vi "TKPS252XG Read Current-Voltage24.vi"(6 "error in (no error)":errorcluster, 8 "channel (ch1:0)":u16(ring) items=["channel 1", "channel 2", "channel 3"], 9 "VISA session":refnum<visa-resource-name>) -> (0 "error out":errorcluster, 1 "voltage limit":dbl format="%.4f", 2 "actual output voltage":dbl format="%.4f", 3 "dup VISA session":refnum<visa-resource-name>, 4 "current limit":dbl format="%.3f", 5 "actual output current":dbl format="%.4f", 7 "output":bool)   [LabVIEW 2024]
doc: "This vi queries the power supply for the current and voltage limits, the actual current and voltage being output, and the output state (on/off)."
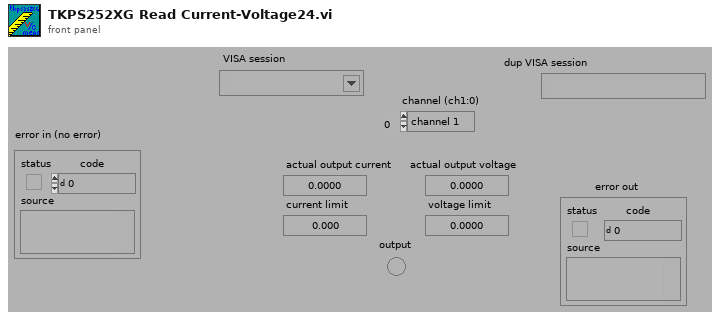
[diagram p1: front panel]
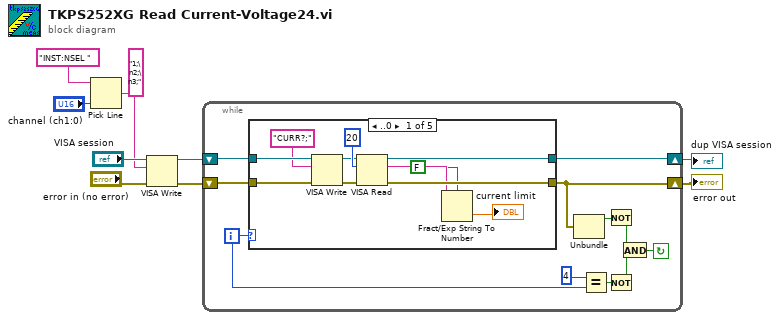
[diagram p0: block diagram]
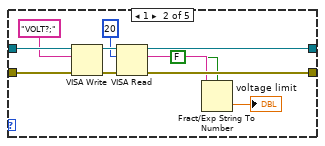
[diagram p2: hidden frame]
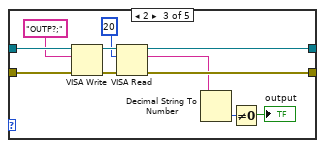
[diagram p3: hidden frame]
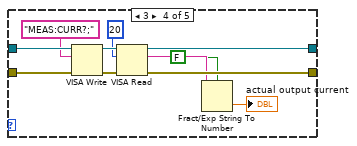
[diagram p4: hidden frame]
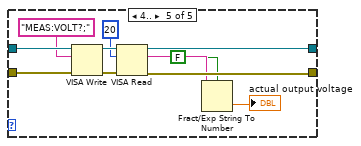
[diagram p5: hidden frame]
diagram:
  n1 = Pick Line(string ("")="INST:NSEL " ("VI name"), multi-line string="1;\n2;\n3;" ("VI name"), line index="channel (ch1:0)") -> (output string=w1:string)
  n2 = VISA Write(VISA resource name="VISA session", write buffer=w1, error in (no error)="error in (no error)") -> (VISA resource name out=w8:refnum<visa-resource-name>, error out=w7:errorcluster)  [unwired: 1 out]
  n3 = while {
    shift-left: w8 -> [w14]
    shift-right: [w12] -> w9
    shift-left: w7 -> [w13]
    shift-right: [w11] -> w10
    i -> [w15]
    stop <- w16 continue-if-true
    n4 = case shown="..0" w15 {
      tunnel: w13 -> [w29 w42 w53 w64 w74]
      tunnel: w14 -> [w28 w41 w52 w63 w73]
      tunnel: [w27 w40 w51 w62 w72] -> w11
      tunnel: [w26 w39 w50 w56 w71] -> w12
      frame ..0 {
        (unwired) FALSE ("use system decimal point (T)")
        n5 = VISA Write(VISA resource name=w28, write buffer="CURR?;", error in (no error)=w29) -> (VISA resource name out=w23:refnum<visa-resource-name>, error out=w32:errorcluster)  [unwired: 1 out]
        n6 = VISA Read(VISA resource name=w23, byte count=u32 20, error in (no error)=w32) -> (VISA resource name out=w26:refnum<visa-resource-name>, read buffer=w25:string, error out=w27:errorcluster)  [unwired: 1 out]
        n7 = Fract/Exp String To Number(use system decimal point (T)=FALSE, string=w25) -> (number=→"current limit":dbl)  [unwired: 2 in, 1 out]
      }
      frame 1 {
        (unwired) FALSE ("use system decimal point (T)")
        n8 = VISA Write(VISA resource name=w41, write buffer="VOLT?;", error in (no error)=w42) -> (VISA resource name out=w35:refnum<visa-resource-name>, error out=w43:errorcluster)  [unwired: 1 out]
        n9 = VISA Read(VISA resource name=w35, byte count=20, error in (no error)=w43) -> (VISA resource name out=w39:refnum<visa-resource-name>, read buffer=w38:string, error out=w40:errorcluster)  [unwired: 1 out]
        n10 = Fract/Exp String To Number(use system decimal point (T)=FALSE, string=w38) -> (number=→"voltage limit":dbl)  [unwired: 2 in, 1 out]
      }
      frame 2 {
        n11 = VISA Write(VISA resource name=w52, write buffer="OUTP?;", error in (no error)=w53) -> (VISA resource name out=w45:refnum<visa-resource-name>, error out=w54:errorcluster)  [unwired: 1 out]
        n12 = VISA Read(VISA resource name=w45, byte count=20, error in (no error)=w54) -> (VISA resource name out=w50:refnum<visa-resource-name>, read buffer=w46:string, error out=w51:errorcluster)  [unwired: 1 out]
        n13 = Decimal String To Number(string=w46) -> (number=w47:i32)  [unwired: 2 in, 1 out]
        n14 = Not Equal To 0?(x=w47) -> (x != 0?=→"output":bool)
      }
      frame 3 {
        (unwired) FALSE ("use system decimal point (T)")
        n15 = VISA Write(VISA resource name=w63, write buffer="MEAS:CURR?;", error in (no error)=w64) -> (VISA resource name out=w58:refnum<visa-resource-name>, error out=w65:errorcluster)  [unwired: 1 out]
        n16 = VISA Read(VISA resource name=w58, byte count=20, error in (no error)=w65) -> (VISA resource name out=w56:refnum<visa-resource-name>, read buffer=w61:string, error out=w62:errorcluster)  [unwired: 1 out]
        n17 = Fract/Exp String To Number(use system decimal point (T)=FALSE, string=w61) -> (number=→"actual output current":dbl)  [unwired: 2 in, 1 out]
      }
      frame 4.. {
        (unwired) FALSE ("use system decimal point (T)")
        n18 = VISA Write(VISA resource name=w73, write buffer="MEAS:VOLT?;", error in (no error)=w74) -> (VISA resource name out=w75:refnum<visa-resource-name>, error out=w76:errorcluster)  [unwired: 1 out]
        n19 = VISA Read(VISA resource name=w75, byte count=20, error in (no error)=w76) -> (VISA resource name out=w71:refnum<visa-resource-name>, read buffer=w70:string, error out=w72:errorcluster)  [unwired: 1 out]
        n20 = Fract/Exp String To Number(use system decimal point (T)=FALSE, string=w70) -> (number=→"actual output voltage":dbl)  [unwired: 2 in, 1 out]
      }
    }
    n21 = Unbundle(w11) -> ("status"=w19:bool)  [unwired: 2 out]
    n22 = Equal?(x=4, y=w15) -> (x = y?=w20:bool)
    n23 = Not(x=w19) -> (.not. x?=w18:bool)
    n24 = Not(x=w20) -> (.not. x?=w17:bool)
    n25 = And(x=w18, y=w17) -> (x .and. y?=w16:bool)
  }
  "error out" <- w10
  "dup VISA session" <- w9
